vi "F Dwf Analog Out Status.vi"(8 "error in (no error)":errorcluster, 10 "idxChannel":i32, 11 "hdwf":i32) -> (0 "error out":errorcluster, 1 "psts":u8, 2 "DwfState":T1(ring), 3 "function return":i32)   [LabVIEW 2019, in "Olasdwf.lvlib"]
doc: "DWFAPI int FDwfAnalogOutStatus(HDWF hdwf, int idxChannel, DwfState *psts);"
uses:
  Olasdwf.lvlib
  Windows/System32/dwf.dll
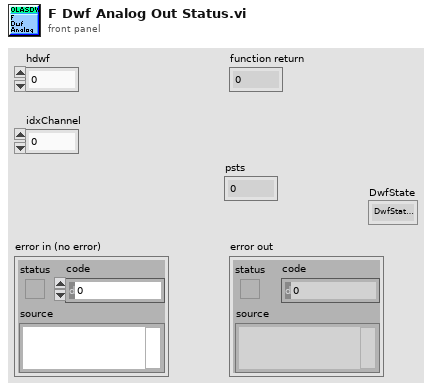
[diagram p1: front panel]
types:
  T1 = enum16{"DwfStateReady", "DwfStateArmed", "DwfStateDone", "DwfStateRunning", "DwfStateTriggered", "DwfStateConfig", "DwfStatePrefill", "DwfStateWait"}
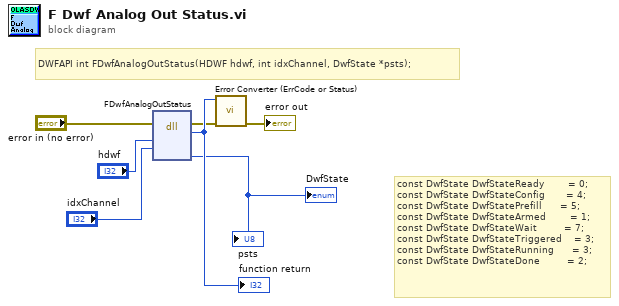
[diagram p0: block diagram]
diagram:
  # "const DwfState DwfStateReady        = 0;\nconst DwfState DwfStateConfig       = 4;\nconst DwfState DwfStatePrefill      = 5;\nconst DwfState DwfStateArmed        = 1;\nconst DwfState DwfStateWait         = 7;\nconst DwfState DwfStateTriggered    = 3;\nconst DwfState DwfStateRunning      = 3;\nconst DwfState DwfStateDone         = 2;"
  # "DWFAPI int FDwfAnalogOutStatus(HDWF hdwf, int idxChannel, DwfState *psts);"
  n1 = dll-call lib="C:/Windows/System32/dwf.*" fn="FDwfAnalogOutStatus"(error in="error in (no error)", "hdwf"="hdwf", "idxChannel"="idxChannel") -> (error out=w3:errorcluster, "return type"=w7:i32, "psts"=→"psts" →"DwfState":u8)  [unwired: 5 in, 1 out]
  "function return" <- w7
  n2 = call "Error Converter (ErrCode or Status).vi"("error in (no error)"=w3, "error code"=w7) -> ("error out"=→"error out":errorcluster)  [unwired: 9 in]
